vi "Main System Model.vi"() -> ()   [LabVIEW 2020]
uses:
  Pump Phases.ctl
  State Machine.ctl
  <vilib>/Utility/file.llb/Read Delimited Spreadsheet (string).vi
  <vilib>/Utility/file.llb/Write Delimited Spreadsheet (string).vi
panel:
  in  "stop 2":bool
  in  "Units":string(combo)="mm"
  in  "Upload Phases":bool
  in  "Path":path
  in  "Save Phases":bool
  in  "State?":bool
  in  "Enum":T1=enum."Delete Unselected"
  in  "Update":bool
  out "Busy":bool
  out "Done":bool[](array[boolean])
  out "Time":timestamp=timestamp(3688120494.225 s since 1904-01-01)
  out "Elapsed Time (s)":dbl
  in  "RUN":bool
  in  "Add":bool
  in  "Pump Phases":T2[](array[typedef]) {"Valve Position" min=0 max=10 step=1; "Pump Rate" format="%#_4g"}
  in  "stop":bool
  in  "Delete last":bool
  in  "Delete unselected":bool
  in  "Show?":bool[](array[boolean])=[TRUE, TRUE, TRUE, TRUE, TRUE, TRUE, TRUE, TRUE, TRUE, TRUE, TRUE, TRUE, TRUE]
  # "SIMULATION MODEL"
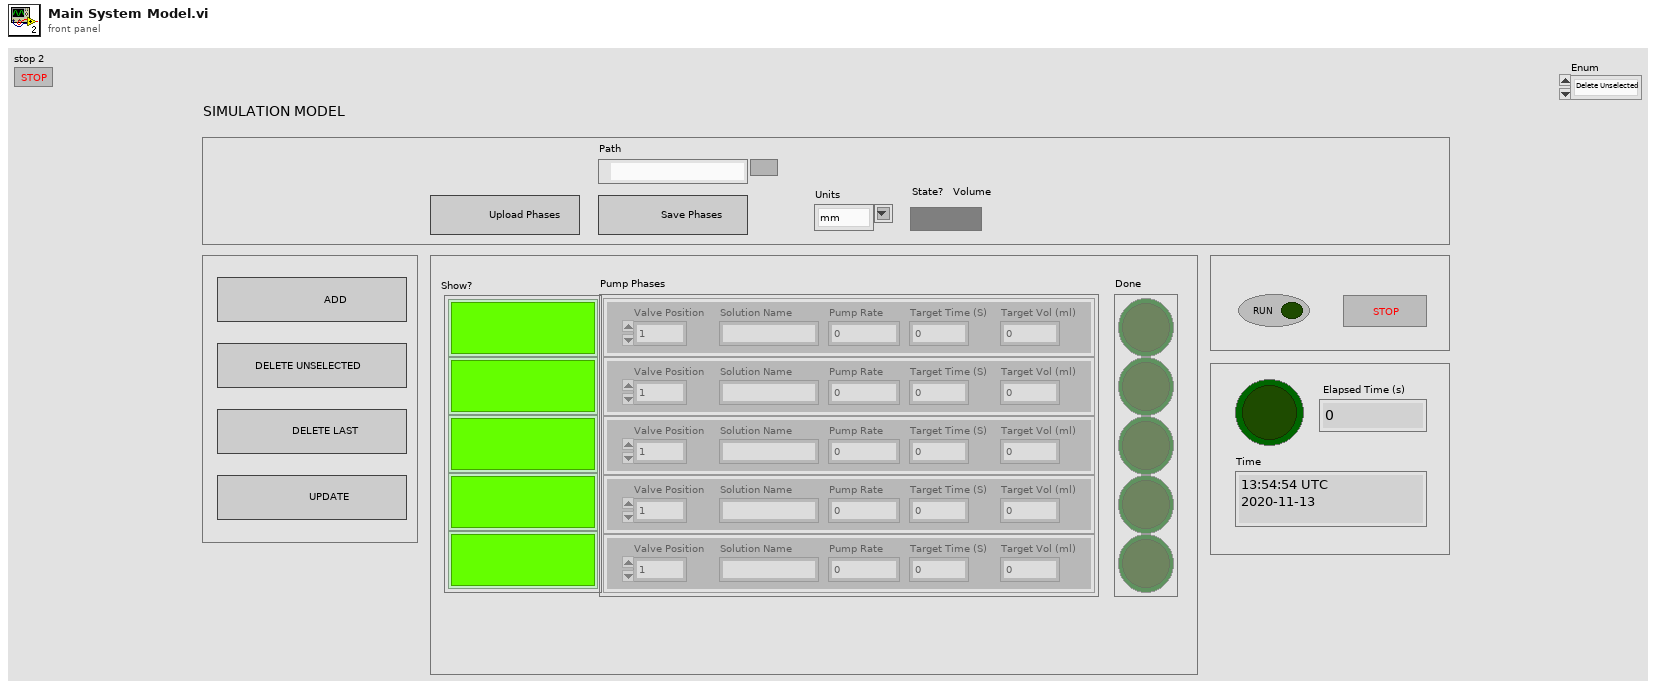
[diagram p1: front panel]
types:
  T1 = typedef "State Machine.ctl" = enum16{"Idle", "Update", "Save Phases", "Upload Phases", "Run", "State", "Delete Unselected", "Add", "Delete Last", "Stop"}
  T2 = typedef "Pump Phases.ctl" = cluster{"Valve Position":sgl, "Solution Name":string, "Pump Rate":dbl, "Target Time":dbl, "Target Volume":dbl}
  T3 = enum8{"Enabled", "Disabled", "Disabled and Grayed Out"}
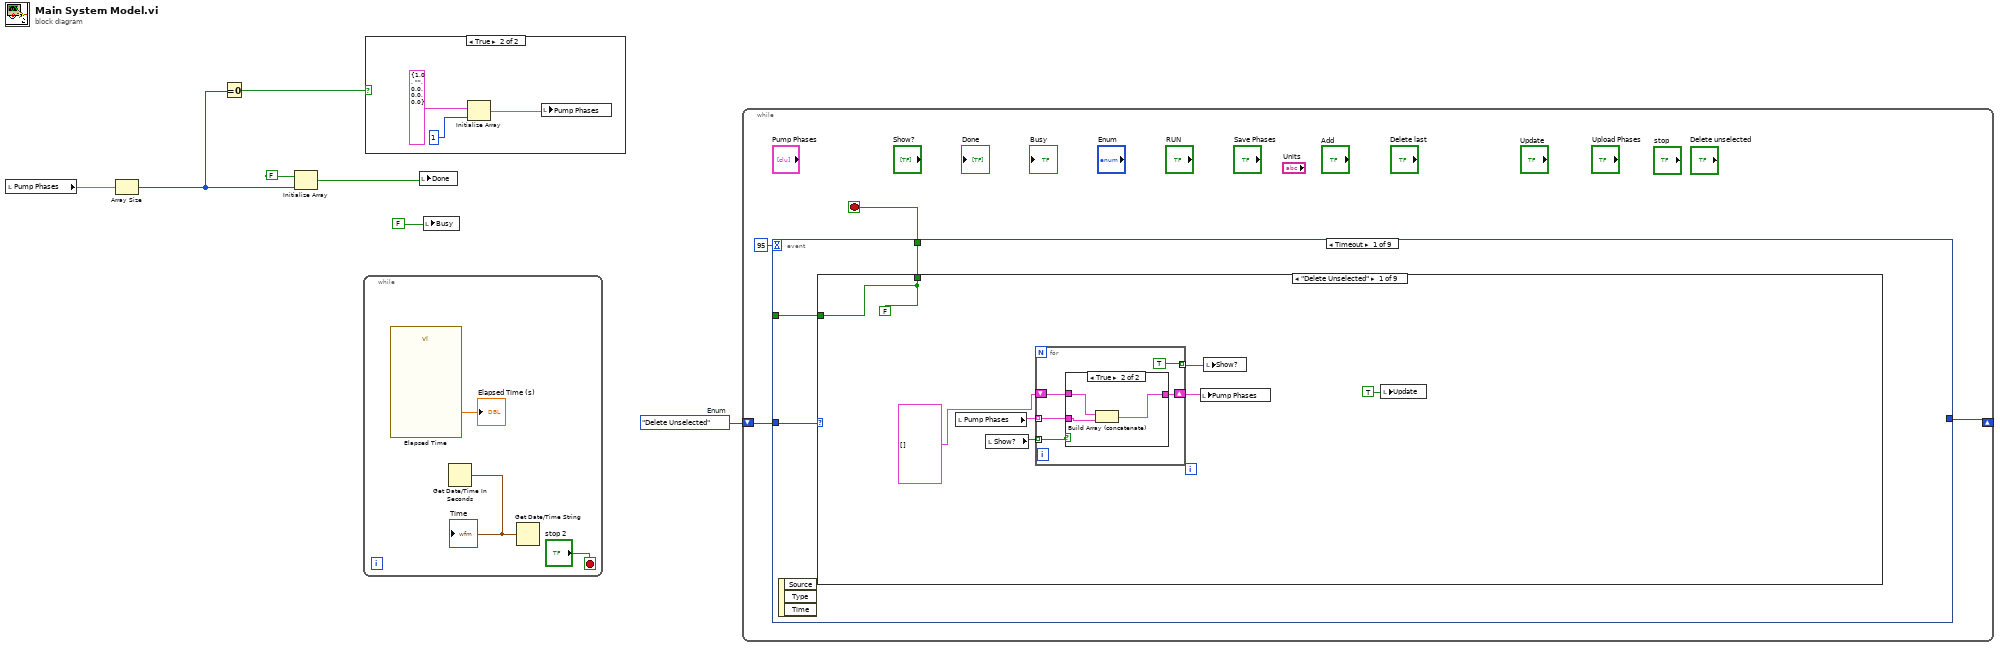
[diagram p0: block diagram]
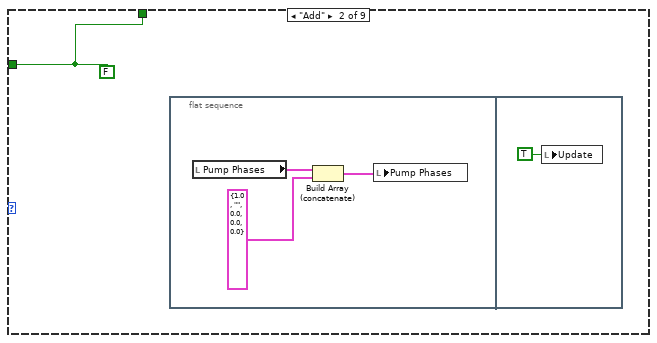
[diagram p4: hidden frame]
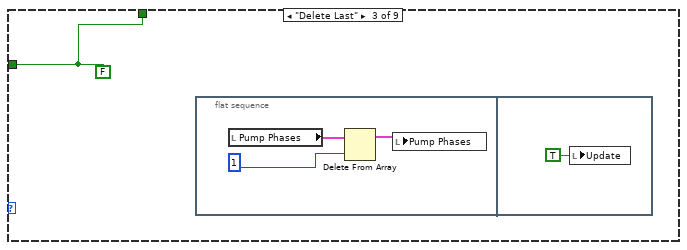
[diagram p5: hidden frame]
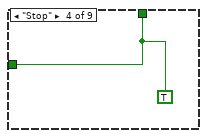
[diagram p6: hidden frame]
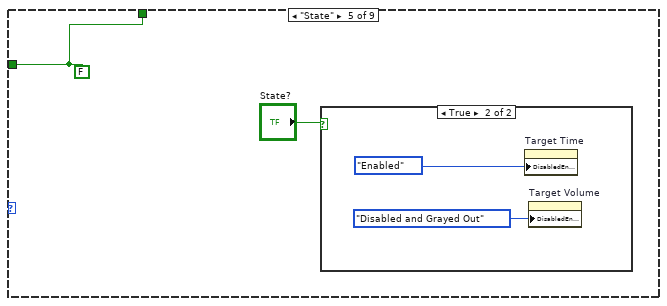
[diagram p7: hidden frame]
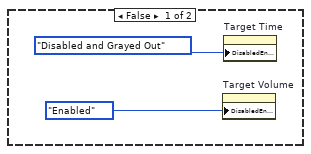
[diagram p8: hidden frame]
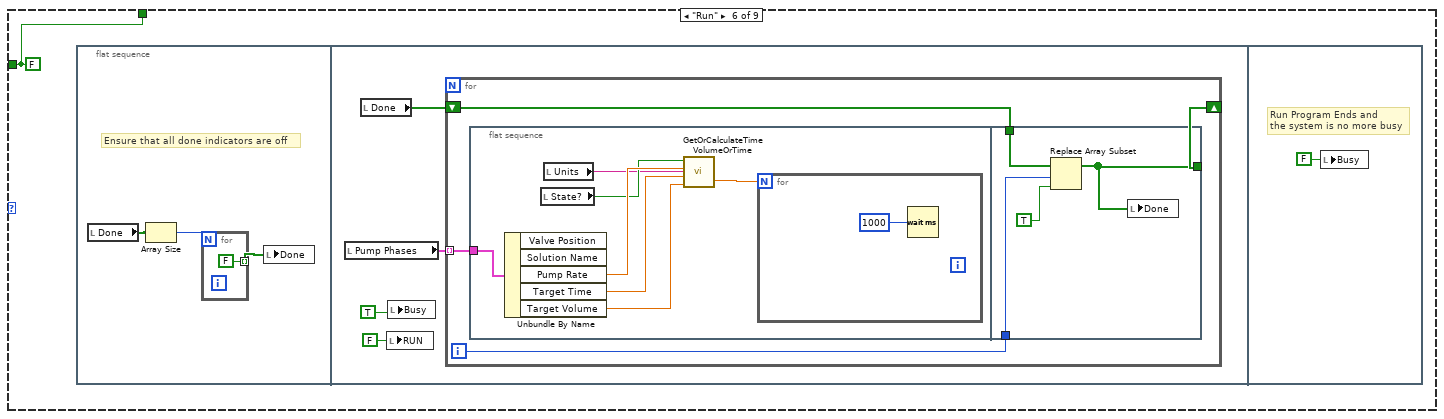
[diagram p9: hidden frame]
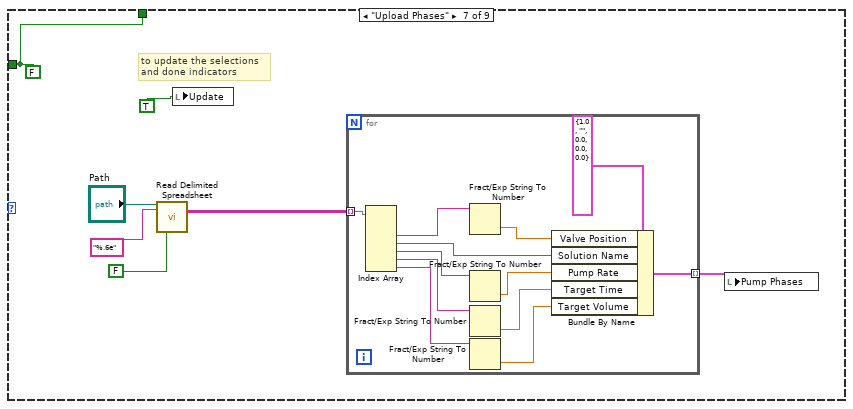
[diagram p10: hidden frame]
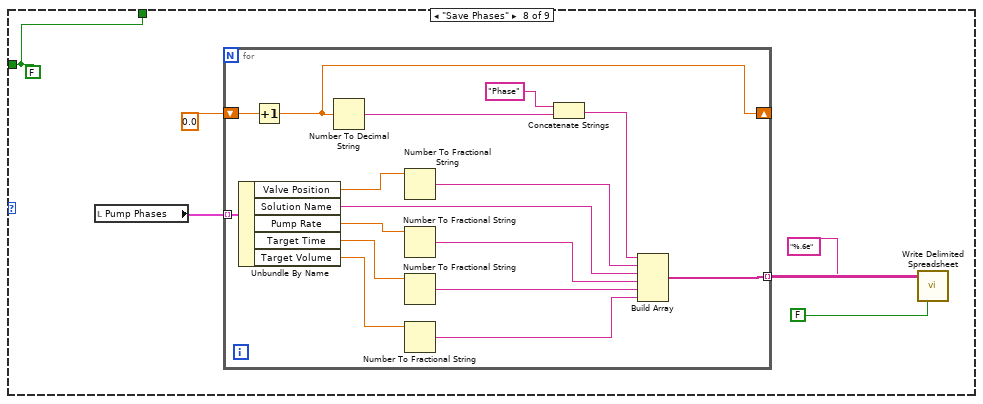
[diagram p11: hidden frame]
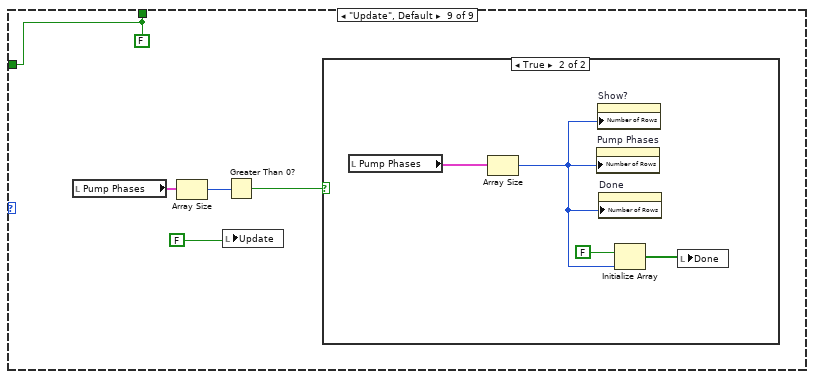
[diagram p12: hidden frame]
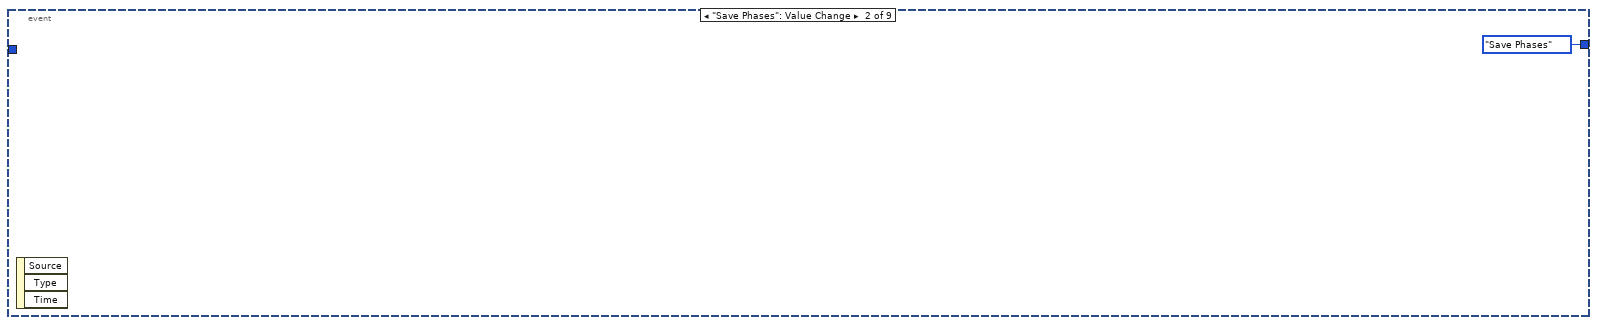
[diagram p14: hidden frame]
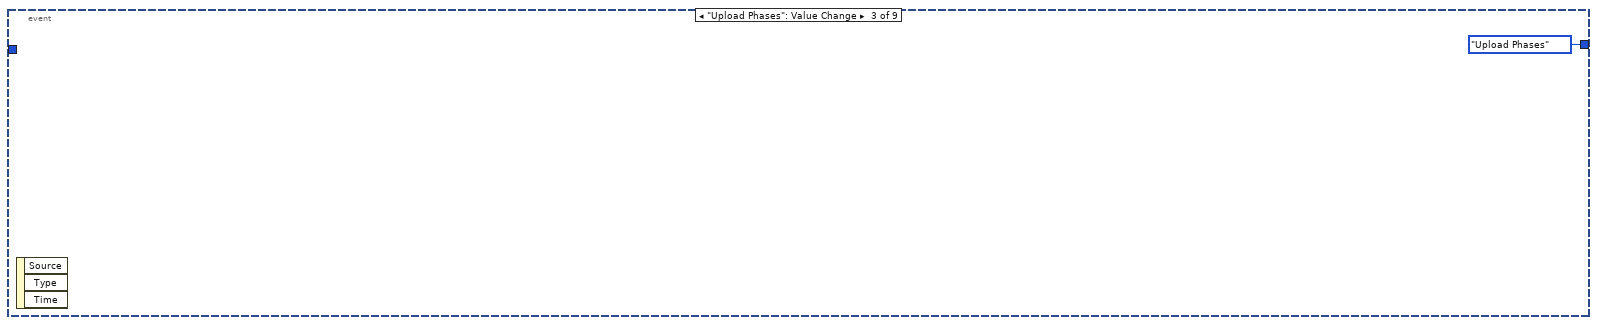
[diagram p15: hidden frame]
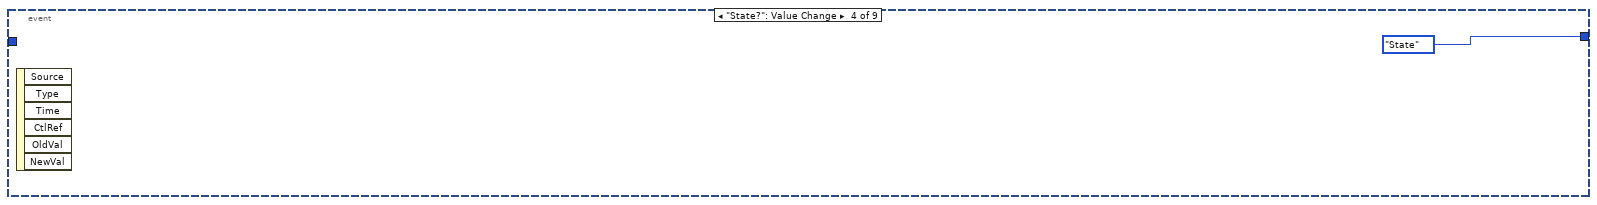
[diagram p16: hidden frame]
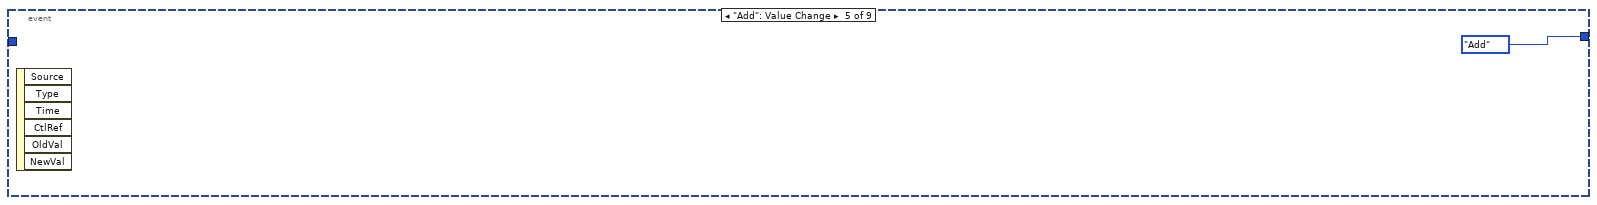
[diagram p17: hidden frame]
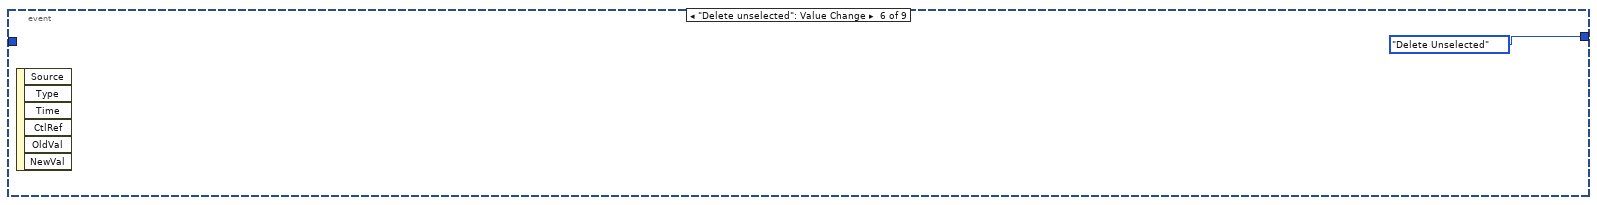
[diagram p18: hidden frame]
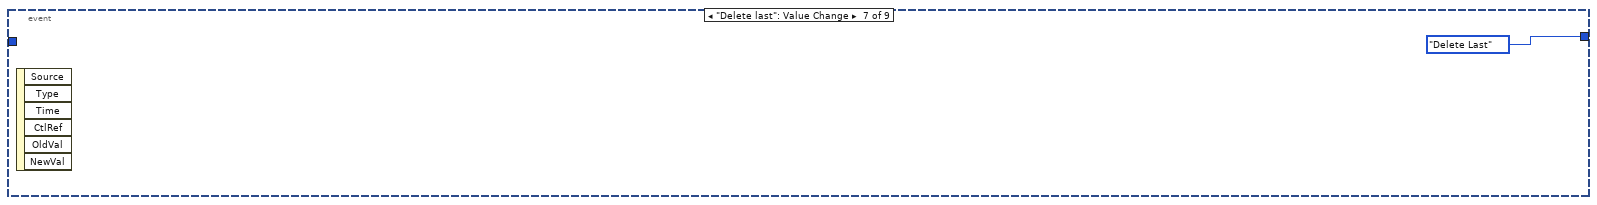
[diagram p19: hidden frame]
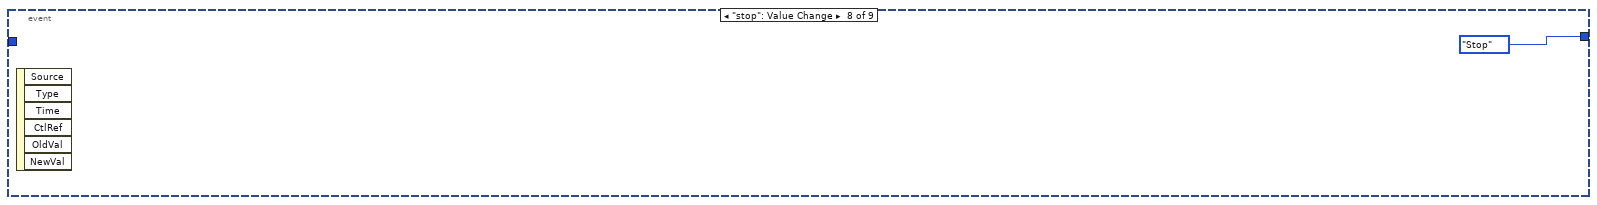
[diagram p20: hidden frame]
diagram:
  w2 = State_Machine."Delete Unselected"  # Enum
  n1 = local read "Pump Phases"() -> (w6:T2[])
  n2 = Array Size(array=w6) -> (size(s)=w4:i32)
  n3 = Equal To 0?(x=w4) -> (x = 0?=w3:bool)
  n4 = Initialize Array "Initialize Array"(FALSE, w4) -> (w7:bool[])
  n5 = while {
    stop <- "stop 2" stop-if-true
    n6 = call "Elapsed Time"() -> ("Elapsed Time (s)"=→"Elapsed Time (s)":dbl)  [unwired: 12 in, 7 out]
    n7 = Get Date/Time In Seconds() -> (seconds since 1Jan1904=w10:timestamp)
    "Time" <- w10
    n8 = Get Date/Time String(seconds (now)=w10) -> ()  [unwired: 2 in, 2 out]
  }
  n9 = case shown="True" w3 {
    frame False {
    }
    frame True {
      n10 = Initialize Array "Initialize Array"(T2 {"Valve Position"=1.0, "Solution Name"="", "Pump Rate"=0.0, "Target Time"=0.0, "Target Volume"=0.0} ("Cluster"), 1 ("dimension size")) -> (w11:T2[])
      n11 = local write "Pump Phases"(w11) -> ()
    }
  }
  n12 = local write "Done"(w7) -> ()
  n13 = local write "Busy"(FALSE) -> ()
  n14 = while {
    shift-right: [w16] -> _
    shift-left: w2 -> [w17]
    stop <- w14 stop-if-true
    n15 = event shown="[0] Timeout" {
      selector: _ -> [_ _ _ _ _ _ _ _ _]
      dyn-events: _ -> [_ _ _ _ _ _ _ _ _]
      timeout: 95 -> [_ _ _ _ _ _ _ _ _]
      tunnel: w17 -> [w20 _ _ _ _ _ _ _ _]
      tunnel: [_ State_Machine."Save Phases" ("Enum") State_Machine."Upload Phases" ("Enum") State_Machine."State" ("Enum") State_Machine."Add" ("Enum") State_Machine."Delete Unselected" ("Enum") State_Machine."Delete Last" ("Enum") State_Machine."Stop" ("Enum") State_Machine."Run" ("Enum")] -> w16
      tunnel: [w19 _ _ _ _ _ _ _ _] -> w14
      tunnel: [w18 _ _ _ _ _ _ _ _] -> _
      event Timeout {
        n16 = event-data() -> ()  [unwired: 1 in, 3 out]
        n17 = case shown="\"Delete Unselected\"" w20 {
          tunnel: [w27 w37 w42 w47 w48 w54 w80 w99 w121] -> w19
          tunnel: [w27 w37 w42 w47 w48 w54 w80 w99 w121] -> w18
          frame "Delete Unselected" {
            w27 = FALSE
            n18 = local read "Pump Phases"() -> (w23:T2[])
            n19 = local read "Show?"() -> (w24:bool[])
            n20 = for {
              tunnel: w23 -> [w31] mode=indexing
              tunnel: w24 -> [w32] mode=indexing
              shift-right: [w28] -> w26
              shift-left: T2[] [] -> [w30]
              tunnel: [TRUE] -> w25 mode=indexing
              n21 = case shown="True" w32 {
                tunnel: w31 -> [_ w36]
                tunnel: [w33 w35] -> w28
                tunnel: w30 -> [w33 w34]
                frame False {
                }
                frame True {
                  n22 = Build Array (concatenate) "Build Array"(w34, w36) -> (w35:T2[])
                }
              }
            }
            n23 = local write "Pump Phases"(w26) -> ()
            n24 = local write "Show?"(w25) -> ()
            n25 = local write "Update"(TRUE) -> ()
          }
          frame "Add" {
            w37 = FALSE
            n26 = flat-sequence {
              frame #0 {
                n27 = local read "Pump Phases"() -> (w40:T2[])
                n28 = Build Array (concatenate) "Build Array"(w40, T2 {"Valve Position"=1.0, "Solution Name"="", "Pump Rate"=0.0, "Target Time"=0.0, "Target Volume"=0.0} ("Cluster")) -> (w39:T2[])
                n29 = local write "Pump Phases"(w39) -> ()
              }
              frame #1 {
                n30 = local write "Update"(TRUE) -> ()
              }
            }
          }
          frame "Delete Last" {
            w42 = FALSE
            n31 = flat-sequence {
              frame #0 {
                n32 = local read "Pump Phases"() -> (w43:T2[])
                n33 = Delete From Array "Delete From Array"(array=w43, length=1) -> (array with subset deleted=w44:T2[])  [unwired: 1 in, 1 out]
                n34 = local write "Pump Phases"(w44) -> ()
              }
              frame #1 {
                n35 = local write "Update"(TRUE) -> ()
              }
            }
          }
          frame "Stop" {
            w47 = TRUE
          }
          frame "State" {
            w48 = FALSE
            n36 = case shown="True" "State?" {
              frame False {
                n37 = property on="Target Volume" class="DigNum (strict)"("DisabledEnum"=T3."Enabled" ("Disabled")) -> ()  [unwired: 2 in, 2 out]
                n38 = property on="Target Time" class="DigNum (strict)"("DisabledEnum"=T3."Disabled and Grayed Out" ("Disabled")) -> ()  [unwired: 2 in, 2 out]
              }
              frame True {
                n39 = property on="Target Time" class="DigNum (strict)"("DisabledEnum"=T3."Enabled" ("Disabled")) -> ()  [unwired: 2 in, 2 out]
                n40 = property on="Target Volume" class="DigNum (strict)"("DisabledEnum"=T3."Disabled and Grayed Out" ("Disabled")) -> ()  [unwired: 2 in, 2 out]
              }
            }
          }
          frame "Run" {
            w54 = FALSE
            n41 = flat-sequence {
              frame #0 {
                # "Ensure that all done indicators are off"
                n42 = local read "Done"() -> (w55:bool[])
                n43 = Array Size(array=w55) -> (size(s)=w56:i32)
                n44 = for {
                  N: w56 -> [_]
                  tunnel: [FALSE] -> w57 mode=indexing
                }
                n45 = local write "Done"(w57) -> ()
              }
              frame #1 {
                n46 = local read "Pump Phases"() -> (w61:T2[])
                n47 = local read "Done"() -> (w60:bool[])
                n48 = local write "RUN"(FALSE ("RUN")) -> ()
                n49 = local write "Busy"(TRUE) -> ()
                n50 = for {
                  tunnel: w61 -> [w66] mode=indexing
                  shift-right: [w64] -> _
                  shift-left: w60 -> [w63]
                  i -> [w65]
                  n51 = flat-sequence {
                    tunnel: w66 -> [w73]
                    tunnel: w65 -> [w78]
                    tunnel: [w75] -> w64
                    tunnel: w63 -> [w76]
                    frame #0 {
                      n52 = Unbundle By Name "Unbundle By Name"(w73) -> ("Pump Rate"=w70:dbl, "Target Time"=w71:dbl, "Target Volume"=w72:dbl)  [unwired: 2 out]
                      n53 = local read "State?"() -> (w69:bool)
                      n54 = local read "Units"() -> (w68:string)
                      n55 = call "GetOrCalculateTime VolumeOrTime.vi"("Units"=w68, "Target Volume"=w72, "Target Time"=w71, "Flow Rate"=w70, "State?"=w69) -> ("Time Output"=w67:dbl)
                      n56 = for {
                        N: w67 -> [_]
                        n57 = Wait (ms)(milliseconds to wait=u32 1000) -> ()  [unwired: 1 out]
                      }
                    }
                    frame #1 {
                      n58 = Replace Array Subset "Replace Array Subset"(array=w76, new element=TRUE, index=w78) -> (w75:bool[])
                      n59 = local write "Done"(w75) -> ()
                    }
                  }
                }
              }
              frame #2 {
                # "Run Program Ends and \nthe system is no more busy"
                n60 = local write "Busy"(FALSE ("Busy")) -> ()
              }
            }
          }
          frame "Upload Phases" {
            w80 = FALSE
            # "to update the selections \nand done indicators"
            n61 = call-poly <vilib>:"Read Delimited Spreadsheet.vi"("file path (dialog if empty)"="Path", "format (%s)"="%.6e" ("format (%.3f)"), "transpose? (F)"=FALSE ("transpose? (no:F)")) -> ("all rows"=w83:string[][])  [unwired: 7 in, 5 out]
            n62 = local write "Update"(TRUE) -> ()
            n63 = for {
              tunnel: w83 -> [w98] mode=indexing
              tunnel: [w90] -> w84 mode=indexing
              n64 = Index Array "Index Array"(array=w98) -> (element #2=w97:string, element #3=w88:string, element #4=w96:string, element #5=w95:string, element #6=w94:string)  [unwired: 6 in, 1 out]
              n65 = Fract/Exp String To Number(string=w97) -> (number=w91:dbl)  [unwired: 3 in, 1 out]
              n66 = Fract/Exp String To Number(string=w96) -> (number=w87:dbl)  [unwired: 3 in, 1 out]
              n67 = Fract/Exp String To Number(string=w95) -> (number=w93:dbl)  [unwired: 3 in, 1 out]
              n68 = Fract/Exp String To Number(string=w94) -> (number=w92:dbl)  [unwired: 3 in, 1 out]
              n69 = Bundle By Name(cluster=T2 {"Valve Position"=1.0, "Solution Name"="", "Pump Rate"=0.0, "Target Time"=0.0, "Target Volume"=0.0} ("Cluster"), "Valve Position"=w91, "Solution Name"=w88, "Pump Rate"=w87, "Target Time"=w93, "Target Volume"=w92) -> (w90:T2)
            }
            n70 = local write "Pump Phases"(w84) -> ()
          }
          frame "Save Phases" {
            w99 = FALSE
            n71 = local read "Pump Phases"() -> (w103:T2[])
            n72 = for {
              tunnel: w103 -> [w110] mode=indexing
              tunnel: [w117] -> w104 mode=indexing
              shift-right: [w113] -> _
              shift-left: 0.0 -> [w112]
              n73 = Unbundle By Name "Unbundle By Name"(w110) -> ("Valve Position"=w107:sgl, "Solution Name"=w108:string, "Pump Rate"=w106:dbl, "Target Time"=w109:dbl, "Target Volume"=w105:dbl)
              n74 = Increment(x=w112) -> (x+1=w113:dbl)
              n75 = Number To Decimal String(number=w113) -> (decimal integer string=w119:string)  [unwired: 1 in]
              n76 = Number To Fractional String(number=w107) -> (F-format string=w111:string)  [unwired: 3 in]
              n77 = Number To Fractional String(number=w106) -> (F-format string=w116:string)  [unwired: 3 in]
              n78 = Number To Fractional String(number=w109) -> (F-format string=w115:string)  [unwired: 3 in]
              n79 = Number To Fractional String(number=w105) -> (F-format string=w114:string)  [unwired: 3 in]
              n80 = Concatenate Strings "Concatenate Strings"("Phase", w119) -> (w118:string)
              n81 = Build Array "Build Array"(w118, w111, w108, w116, w115, w114) -> (w117:string[])
            }
            n82 = call-poly <vilib>:"Write Delimited Spreadsheet.vi"("format (%s)"="%.6e" ("format (%.3f)"), "2D data"=w104, "transpose? (no:F)"=FALSE) -> ()  [unwired: 11 in, 2 out]
          }
          frame "Update", Default {
            w121 = FALSE
            n83 = local read "Pump Phases"() -> (w124:T2[])
            n84 = Array Size(array=w124) -> (size(s)=w123:i32)
            n85 = local write "Update"(FALSE) -> ()
            n86 = Greater Than 0?(x=w123) -> (x > 0?=w125:bool)
            n87 = case shown="True" w125 {
              frame False {
              }
              frame True {
                n88 = local read "Pump Phases"() -> (w129:T2[])
                n89 = Array Size(array=w129) -> (size(s)=w126:i32)
                n90 = property on="Pump Phases" class="Arr (strict)"("Number of Rows"=w126) -> ()  [unwired: 2 in, 2 out]
                n91 = property on="Show?" class="Arr (strict)"("Number of Rows"=w126) -> ()  [unwired: 2 in, 2 out]
                n92 = property on="Done" class="Arr (strict)"("Number of Rows"=w126) -> ()  [unwired: 2 in, 2 out]
                n93 = Initialize Array "Initialize Array"(FALSE, w126) -> (w127:bool[])
                n94 = local write "Done"(w127) -> ()
              }
            }
          }
        }
      }
      event "Save Phases": Value Change {
        n95 = event-data() -> ()  [unwired: 1 in, 3 out]
      }
      event "Upload Phases": Value Change {
        n96 = event-data() -> ()  [unwired: 1 in, 3 out]
      }
      event "State?": Value Change {
        n97 = event-data() -> ()  [unwired: 1 in, 6 out]
      }
      event "Add": Value Change {
        n98 = event-data() -> ()  [unwired: 1 in, 6 out]
      }
      event "Delete unselected": Value Change {
        n99 = event-data() -> ()  [unwired: 1 in, 6 out]
      }
      event "Delete last": Value Change {
        n100 = event-data() -> ()  [unwired: 1 in, 6 out]
      }
      event "stop": Value Change {
        n101 = event-data() -> ()  [unwired: 1 in, 6 out]
      }
      event "RUN": Value Change {
        n102 = event-data() -> ()  [unwired: 1 in, 6 out]
      }
    }
  }
